vi "GPSGGA.vi"(0 "String":string) -> (1 "Altitud":string, 2 "Sep Geoide":string, 3 "Ubicación":string, 4 "Hora":string, 5 "Fix Status":string, 6 "# Satelite":string)   [LabVIEW 2020]
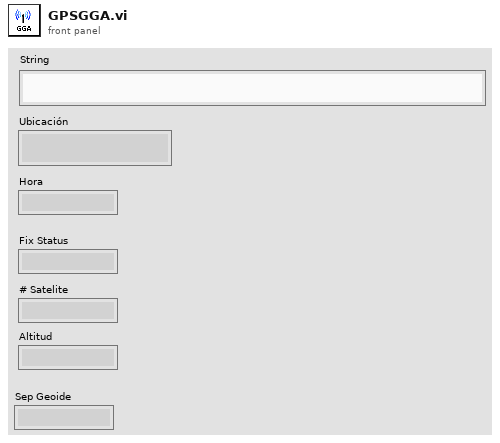
[diagram p1: front panel]
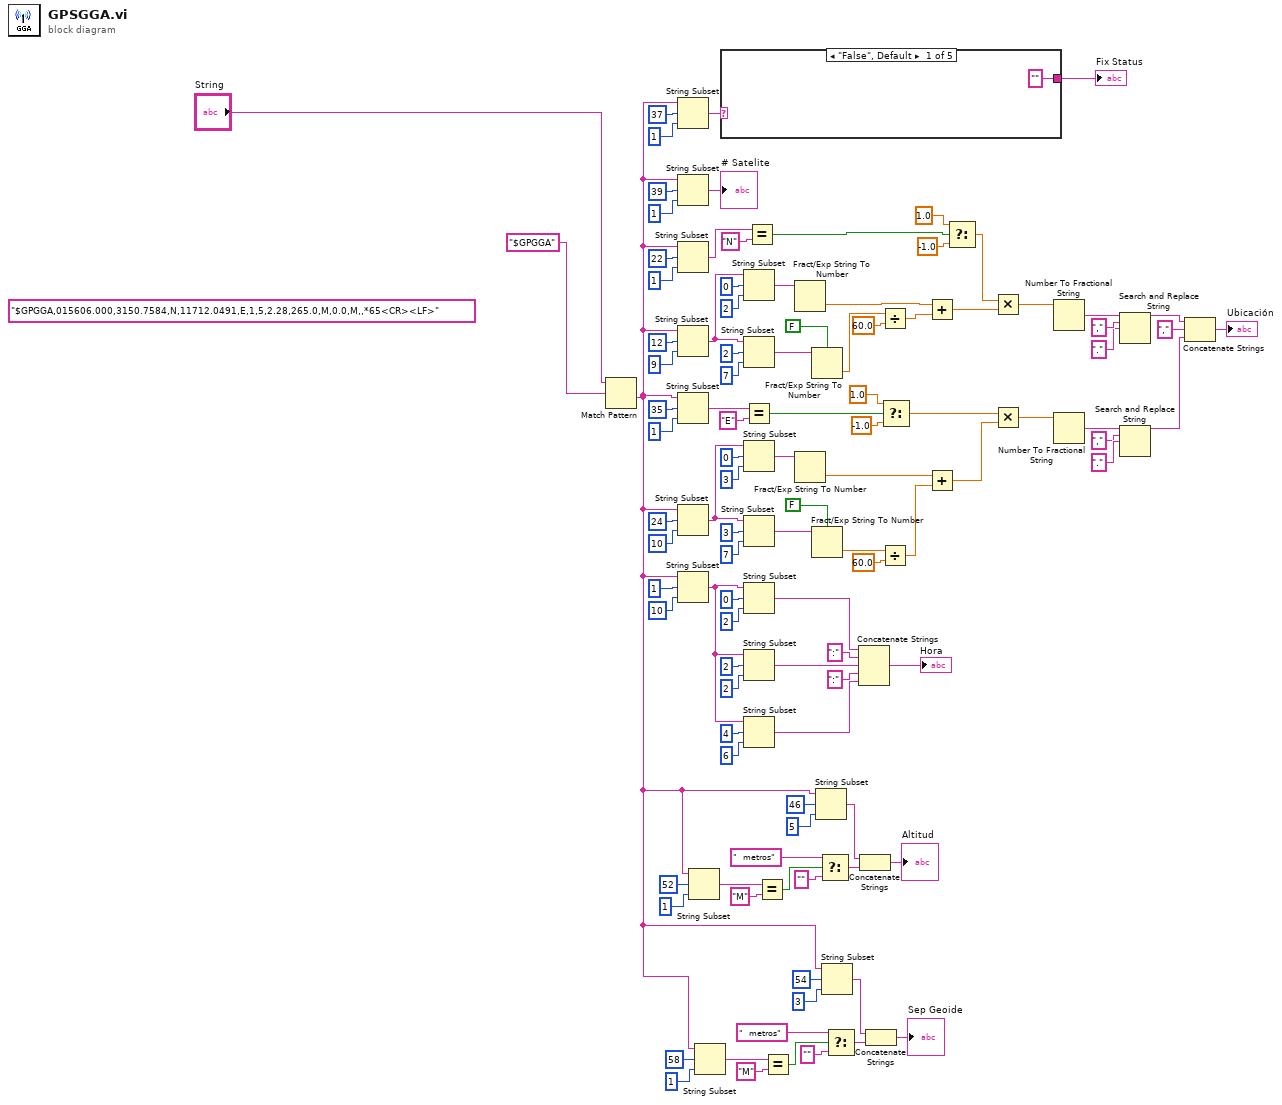
[diagram p0: block diagram]
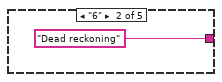
[diagram p2: hidden frame]
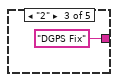
[diagram p3: hidden frame]
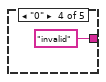
[diagram p4: hidden frame]
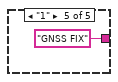
[diagram p5: hidden frame]
diagram:
  (unwired) "$GPGGA,015606.000,3150.7584,N,11712.0491,E,1,5,2.28,265.0,M,0.0,M,,*65<CR><LF>"
  n1 = Match Pattern(string="String", regular expression="$GPGGA") -> (after substring=w2:string)  [unwired: 1 in, 3 out]
  n2 = String Subset(string=w2, offset (0)=37, length (rest)=1 ("length (rest)")) -> (substring=w28:string)
  n3 = String Subset(string=w2, offset (0)=39, length (rest)=1 ("length (rest)")) -> (substring=→"# Satelite":string)
  n4 = String Subset(string=w2, offset (0)=22, length (rest)=1 ("length (rest)")) -> (substring=w88:string)
  n5 = String Subset(string=w2, offset (0)=12, length (rest)=9 ("length (rest)")) -> (substring=w100:string)
  n6 = String Subset(string=w2, offset (0)=35, length (rest)=1 ("length (rest)")) -> (substring=w62:string)
  n7 = String Subset(string=w2, offset (0)=24, length (rest)=10 ("length (rest)")) -> (substring=w72:string)
  n8 = String Subset(string=w2, offset (0)=1, length (rest)=10 ("length (rest)")) -> (substring=w43:string)
  n9 = String Subset(string=w2, offset (0)=52, length (rest)=1 ("length (rest)")) -> (substring=w21:string)
  n10 = String Subset(string=w2, offset (0)=58, length (rest)=1 ("length (rest)")) -> (substring=w8:string)
  n11 = case shown="\"False\", Default" w28 {
    tunnel: ["" "Dead reckoning" "DGPS Fix" "invalid" "GNSS FIX"] -> w27
    frame "False", Default {
    }
    frame "6" {
    }
    frame "2" {
    }
    frame "0" {
    }
    frame "1" {
    }
  }
  "Fix Status" <- w27
  n12 = String Subset(string=w100, offset (0)=0, length (rest)=2 ("length (rest)")) -> (substring=w96:string)
  n13 = String Subset(string=w100, offset (0)=2, length (rest)=7 ("length (rest)")) -> (substring=w97:string)
  n14 = Equal?(x=w62, y="E") -> (x = y?=w64:bool)
  n15 = String Subset(string=w72, offset (0)=0, length (rest)=3 ("length (rest)")) -> (substring=w76:string)
  n16 = String Subset(string=w72, offset (0)=3, length (rest)=7 ("length (rest)")) -> (substring=w75:string)
  n17 = String Subset(string=w43, offset (0)=0, length (rest)=2 ("length (rest)")) -> (substring=w40:string)
  n18 = String Subset(string=w43, offset (0)=2, length (rest)=2 ("length (rest)")) -> (substring=w38:string)
  n19 = String Subset(string=w43, offset (0)=4, length (rest)=6 ("length (rest)")) -> (substring=w36:string)
  n20 = Equal?(x=w88, y="N") -> (x = y?=w86:bool)
  n21 = Equal?(x=w21, y="M") -> (x = y?=w19:bool)
  n22 = Equal?(x=w8, y="M") -> (x = y?=w10:bool)
  n23 = Fract/Exp String To Number(string=w96) -> (number=w92:dbl)  [unwired: 3 in, 1 out]
  n24 = Fract/Exp String To Number(string=w76) -> (number=w80:dbl)  [unwired: 3 in, 1 out]
  n25 = Fract/Exp String To Number(use system decimal point (T)=FALSE, string=w97) -> (number=w94:dbl)  [unwired: 2 in, 1 out]
  n26 = Fract/Exp String To Number(use system decimal point (T)=FALSE, string=w75) -> (number=w78:dbl)  [unwired: 2 in, 1 out]
  n27 = String Subset(string=w2, offset (0)=46, length (rest)=5 ("length (rest)")) -> (substring=w22:string)
  n28 = Select(t="  metros", s=w19, f="") -> (s? t:f=w16:string)
  n29 = String Subset(string=w2, offset (0)=54, length (rest)=3 ("length (rest)")) -> (substring=w7:string)
  n30 = Select(t="  metros", s=w10, f="") -> (s? t:f=w13:string)
  n31 = Concatenate Strings(w40, ":" ("string"), w38, ":" ("string"), w36) -> (→"Hora":string)
  n32 = Concatenate Strings(w22, w16) -> (→"Altitud":string)
  n33 = Concatenate Strings(w7, w13) -> (→"Sep Geoide":string)
  n34 = Divide(x=w94, y=60.0) -> (x/y=w91:dbl)
  n35 = Divide(x=w78, y=60.0) -> (x/y=w81:dbl)
  n36 = Select(t=1.0, s=w64, f=-1.0) -> (s? t:f=w67:dbl)
  n37 = Add(x=w92, y=w91) -> (x+y=w82:dbl)
  n38 = Add(x=w80, y=w81) -> (x+y=w61:dbl)
  n39 = Select(t=1.0, s=w86, f=-1.0) -> (s? t:f=w83:dbl)
  n40 = Multiply(x=w83, y=w82) -> (x*y=w58:dbl)
  n41 = Multiply(x=w67, y=w61) -> (x*y=w57:dbl)
  n42 = Number To Fractional String(number=w58) -> (F-format string=w56:string)  [unwired: 3 in]
  n43 = Number To Fractional String(number=w57) -> (F-format string=w51:string)  [unwired: 3 in]
  n44 = Search and Replace String(input string=w56, search string=",", replace string="." ("replace string (\"\")")) -> (result string=w48:string)  [unwired: 5 in, 3 out]
  n45 = Search and Replace String(input string=w51, search string=",", replace string="." ("replace string (\"\")")) -> (result string=w50:string)  [unwired: 5 in, 3 out]
  n46 = Concatenate Strings(w48, "," ("string"), w50) -> (→"Ubicación":string)
